vi "OE1201_Configure Sine Out.vi"(7 "OE1201_Configure Sine Out":cluster{"Sine Output Amplitude (V)":dbl}={"Sine Output Amplitude (V)"=0.1} {"Sine Output Amplitude (V)" min=0.1 max=1.0 format="%.3f"}, 8 "Error in (no error)":errorcluster caption="error out（no error）", 9 "Remote Mode":u16(ring) items=["USB", "RS232"], 11 "VISA resource name":refnum<visa-resource-name>) -> (0 "Error out":errorcluster caption="error out", 1 "Output String":string, 3 "VISA resource  out":refnum<visa-resource-name>)   [LabVIEW 2011]
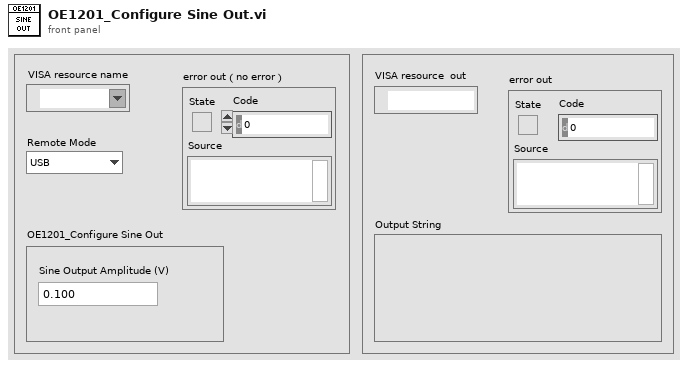
[diagram p1: front panel]
types:
  T1 = enum16{"ISRC", "IGND", "ICPL", "ILIN", "PHAS", "FMOD", "RSLP", "FREQ", "SWPT", "SLLM", "SULM", "SSLL", "SSLG", "STLM", "SWRM", "IRNG", "SENS", "RMOD", "OFLT", "OFSL", "SYNC", "DMOD", "HARM", "DARB", "SWVT", "SLVL", "SVLL", "SVUL", "SVSL", "SVSG", "SVTM", "SVRM", "RALL", "SNAP", "OUTP", "OAUX", "COUT", "CAUX", "COFP", "CEXP", "FPOP", "OEXP", "*IDN", "*RST", "OVLD", "INOV", "GNOV", "*PLL", "SSET", "RSET", "AGAN", "APHS", "ARSV", "ASCL", "EQCD", "EQCS", "SPED", "SRAT", "SLEN", "SSLE", "STRG", "SPRM", "STRD", "PAUS", "REST", "SPTS", "TRCA", "TEMP", "RSTU", "IHNZ", "DEQU", "SADD", "ARNG", "CSPE", "ISRCD", "IGNDD", "ICPLD", "ILIND", "PHASD", "FMODD", "RSLPD", "FREQD", "SWPTD", "SLLMD", "SULMD", "SSLLD", "SSLGD", "STLMD", "SWRMD", "SENSD", "RMODD", "OFLTD", "OFSLD", "SYNCD", "HARMD", "EQCDD", "EQCSD", "SNAPD", "OUTPD", "SWVTD", "SLVLD", "SVLLD", "SVULD", "SVSLD", "SVSGD", "SVTMD", "SVRMD", "SVDCD", "ARSVD", "AGAND", "APHSD", "ASCLD", "FPOPD", "CAUXD", "OEXPD", "SPEDD", "SRATD", "SLEND", "SSLED", "STRGD", "SPRMD", "STRDD", "PAUSD", "RESTD", "SPTSD", "TRCAD", "*IDND", "*RSTD", "INOVD", "GNOVD", "*PLLD", "SSETD", "RSETD"}
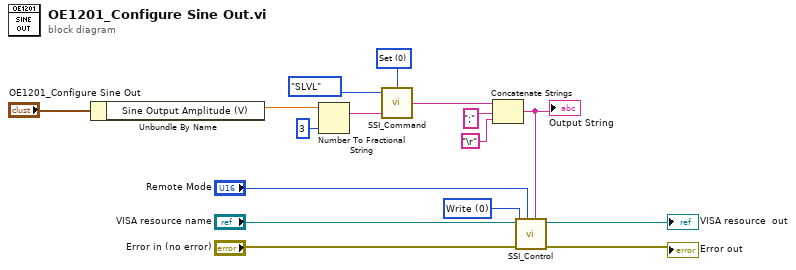
[diagram p0: block diagram]
diagram:
  w5 = u16 0 items=["Set", "Query"] ("Opera")
  w15 = u16 0 items=["Write", "Read"] ("Control")
  n1 = Unbundle By Name("OE1201_Configure Sine Out") -> ("Sine Output Amplitude (V)"=w4:dbl)
  n2 = Number To Fractional String(number=w4, precision (6)=i16 3 ("宽度(-)")) -> (F-format string=w9:string)  [unwired: 2 in]
  n3 = call "SSI_Command.vi"("Opera"=w5, "Paramter"=w9, "Command Type"=T1."SLVL") -> ("Output string"=w6:string)  [unwired: 1 in]
  n4 = Concatenate Strings(w6, ";" ("替换字符串(\"\")"), "\r") -> (w10:string)
  "Output String" <- w10
  n5 = call "SSI_Control.vi"("Write Buffer"=w10, "Remote Mode"="Remote Mode", "Error in (no error)"="Error in (no error)", "Control"=w15, "VISA resource name"="VISA resource name") -> ("Error out"=→"Error out":errorcluster, "VISA resource  out"=→"VISA resource  out":refnum<visa-resource-name>)  [unwired: 3 in, 2 out]
